vi "Legacy_ProdLight MainUI_controls_and_indicators -barebones.vi"() -> ()   [LabVIEW 2017]
panel:
  in  "MoveTowardFast":bool caption="Move \nToward\nFast"
  in  "MoveToZero":bool caption="Move to \nZero"
  in  "MoveAwayFast":bool caption="Move \nAway Fast"
  in  "MoveToward":bool caption="Move \nToward (-)"
  in  "MoveAway":bool caption="Move \nAway (+)"
  out "Safety OK":bool
  in  "SystemError":bool
  out "Pos Err (cnts)":dbl
  out "MotorPos(in)":dbl caption="Motor Position (in)" format="%.3f"
  in  "StatusMsg":string caption="Status"
  in  "Weld Enable":bool caption="Weld Current\nSetpoint"
  out "JoggingTurntable":bool
  in  "JogTurntable":bool caption="Click and Hold"
  out "SeqLoaded":bool caption="Sequence Loaded"
  out "SeqAborted":bool caption="Sequence Aborted"
  in  "AbortSeq":bool
  in  "MotorCtrlLoop Enable":bool caption="Motor Pos\nLoop Ctrl"
  in  "Turntable Enable":bool caption="Turntable On"
  out "SeqRunning":bool
  in  "StartSeq":bool
  out "Sequence File":string
  in  "Tab Control":enum32{"Config", "Data", "Motor", "Seq"}(tab)
  in  "IgnoreMtrRspnsErr":bool caption="Ignore Motor\nResponse Error\nDuring Seq"
  in  "AVC ConfigUtility":bool caption="AVC Configuration\nUtility"
  in  "SamplingRate":dbl=1000.0 caption="Sampling\nRate"
  in  "NumSamples":i32=100 caption="Samples per\nAcquistion"
  in  "UpdateDAQSettings":bool
  in  "DAQ Rd & MtrSP Interval":u32
  in  "WriteLogFile Interval":u32
  in  "DAQDisplay Interval":i32
  out "DAQEnabled":bool
  in  "DAQEnDis":bool
  out "LogEnabled":bool
  in  "LogEnDis":bool
  out "TDMSEnabled":bool
  in  "TDMSEnDis":bool
  in  "PosCtlrSettings":bool caption="Position Ctlr\nRunTime Settings"
  out "MotorRspnsErr":bool caption="Motor Response\nError"
  out "TotalVgain":dbl caption="Total Ctlr\nVgain" format="%.3f"
  out "Motor SP":dbl caption="Computed Motor\nPos Chg (in)" format="%.3f"
  out "VoltageError":dbl caption="Voltage Error" format="%.3f"
  out "WeldTime":dbl caption="Weld Time (s)" format="%.2f"
  out "voltage fb":dbl caption="Voltage" format="%.3f"
  out "Current SP":dbl format="%.3f"
  out "Current fb":dbl caption="Current" format="%.3f"
  out "ProcessTime":dbl caption="Process Time (s)" format="%.2f"
  out "AVC Lockout":bool
  out "In Range?":bool
  out "VspOffset":dbl
  out "Volts and Current Chart":T1(graph)
  in  "GraphEnable":bool
  out "DAQ Latency":bool caption="Time has Elapsed"
  out "SeqList":i32(listbox) caption="Sequence"
  out "Step Comment":string
  in  "Turntable \nSpeed (RPM)":dbl(knob) scale=0.0..10.0
  out "Process Complete":bool caption="Time has Elapsed"
  out "Weld Profile Graph":cluster{dbl[], dbl[]}(graph)
  out "Weld Current Waveform Chart":dbl(graph)
  in  "Exit":bool
  in  "AbortSeq - NonLatchingCtrl":bool
  # "Configuration Panel"
  # "DAQ Settings"
  # "Run Time Data Panel"
  # "V & I Process Feedback"
  # "click to reset"
  # "Voltage FB (V)"
  # "Current FB (A)"
  # "Motor Pos (in)"
  # "Right-Click to Clear"
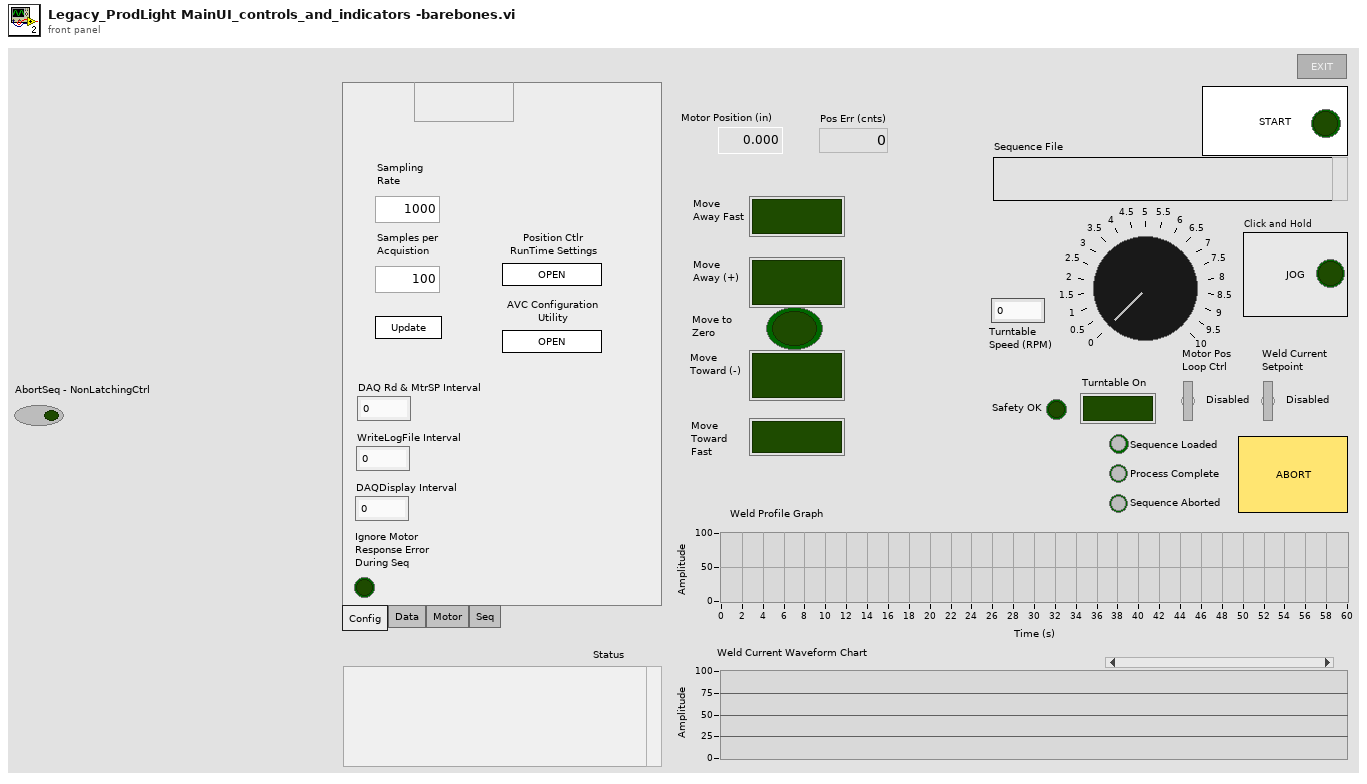
[diagram p1: front panel]
types:
  T1 = cluster{"VoltageDyn":dbl, "CurrentDyn":dbl, "MotorV SP":dbl}
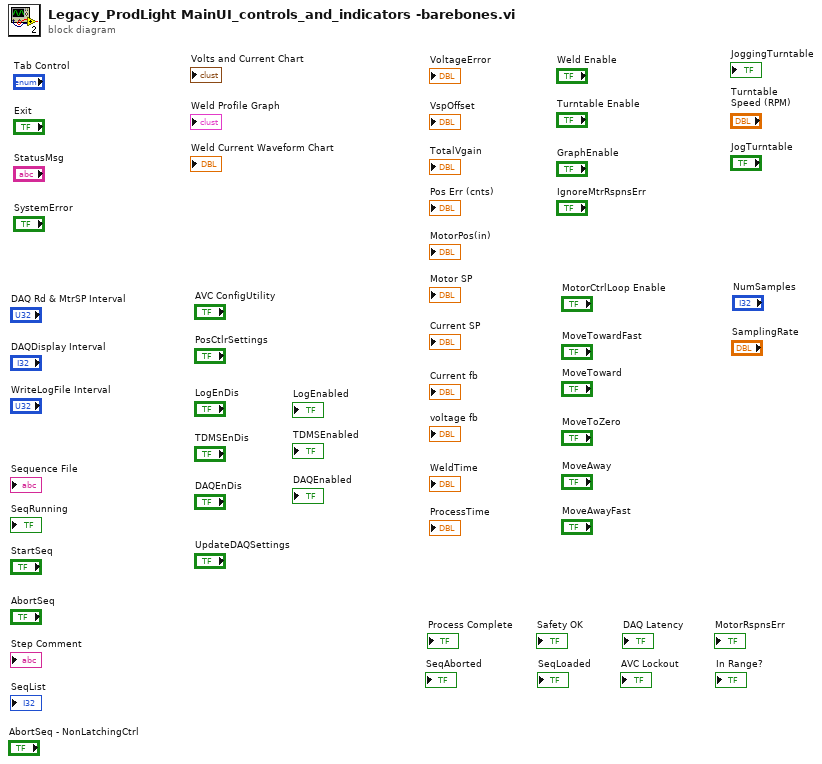
[diagram p0: block diagram]
diagram:
